vi "UI_ctrl_fgv.vi"(7 "cmd":T2, 11 "UI cluster in":T1) -> (3 "UI cluster out":T1)   [LabVIEW 2016]
uses:
  ctl/UI_cmd-ctl.ctl
  ctl/UI_ctl.ctl
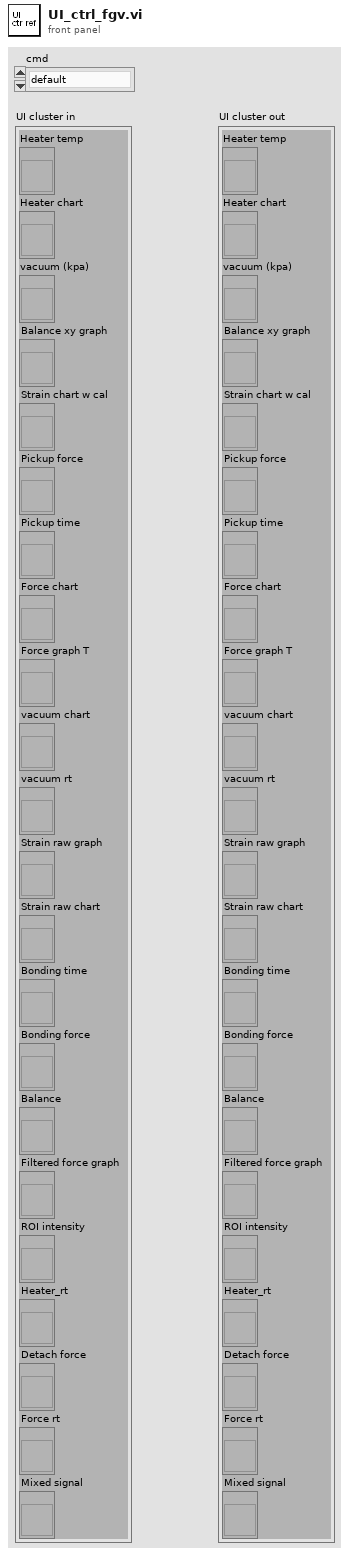
[diagram p1: front panel]
types:
  T1 = typedef "UI_ctl.ctl" = cluster{"Heater temp":refnum<vi>, "Heater chart":refnum<vi>, "vacuum (kpa)":refnum<vi>, "Balance xy graph":refnum<vi>, "Strain chart w cal":refnum<vi>, "Pickup force":refnum<vi>, "Pickup time":refnum<vi>, "Force chart":refnum<vi>, "Force graph T":refnum<vi>, "vacuum chart":refnum<vi>, "vacuum rt":refnum<vi>, "Strain raw graph":refnum<vi>, "Strain raw chart":refnum<vi>, "Bonding time":refnum<vi>, "Bonding force":refnum<vi>, "Balance":refnum<vi>, "Filtered force graph":refnum<vi>, "ROI intensity":refnum<vi>, "Heater_rt":refnum<vi>, "Detach force":refnum<vi>, "Force rt":refnum<vi>, "Mixed signal":refnum<vi>}
  T2 = typedef "UI_cmd-ctl.ctl" = enum16{"default", "create", "read"}
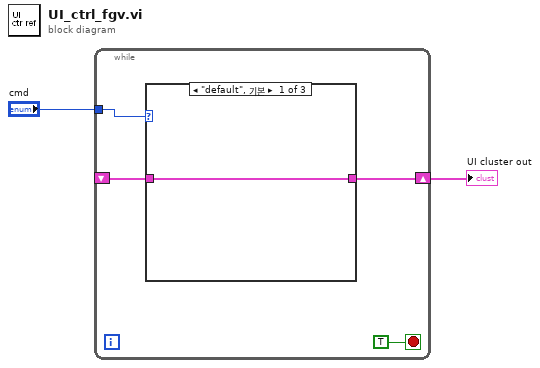
[diagram p0: block diagram]
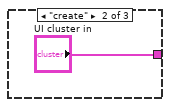
[diagram p2: hidden frame]
diagram:
  n1 = while {
    tunnel: "cmd" -> [w6]
    shift-right: [w4] -> w1
    shift-left: _ -> [w3]
    stop <- TRUE stop-if-true
    n2 = case shown="\"default\", 기본" w6 {
      tunnel: [w7 "UI cluster in" w9] -> w4
      tunnel: w3 -> [w7 _ w9]
      frame "default", Default {
      }
      frame "create" {
      }
      frame "read" {
      }
    }
  }
  "UI cluster out" <- w1
